vi "대한상공회의소 데이터셋 모으기(SM).vi"() -> ()   [LabVIEW 2020]
uses:
  <vilib>/DAQmx/read.llb/DAQmx Read (Analog 1D Wfm NChan NSamp).vi
  <vilib>/Analysis/baseanly.llb/Mean (DBL).vi
  <vilib>/DAQmx/create/channels.llb/DAQmx Create Channel (AI-Voltage-Basic).vi
  <vilib>/DAQmx/configure/timing.llb/DAQmx Timing (Sample Clock).vi
  <vilib>/DAQmx/miscellaneous.llb/DAQmx Fill In Error Info.vi
  <vilib>/Utility/file.llb/Write Delimited Spreadsheet (DBL).vi
  <vilib>/Analysis/NI_AALBase.lvlib
panel:
  in  "저장":bool
  out "결과":string
  out "출력 클러스터":cluster{dbl, dbl, dbl, dbl}(graph)
  in  "정지":bool
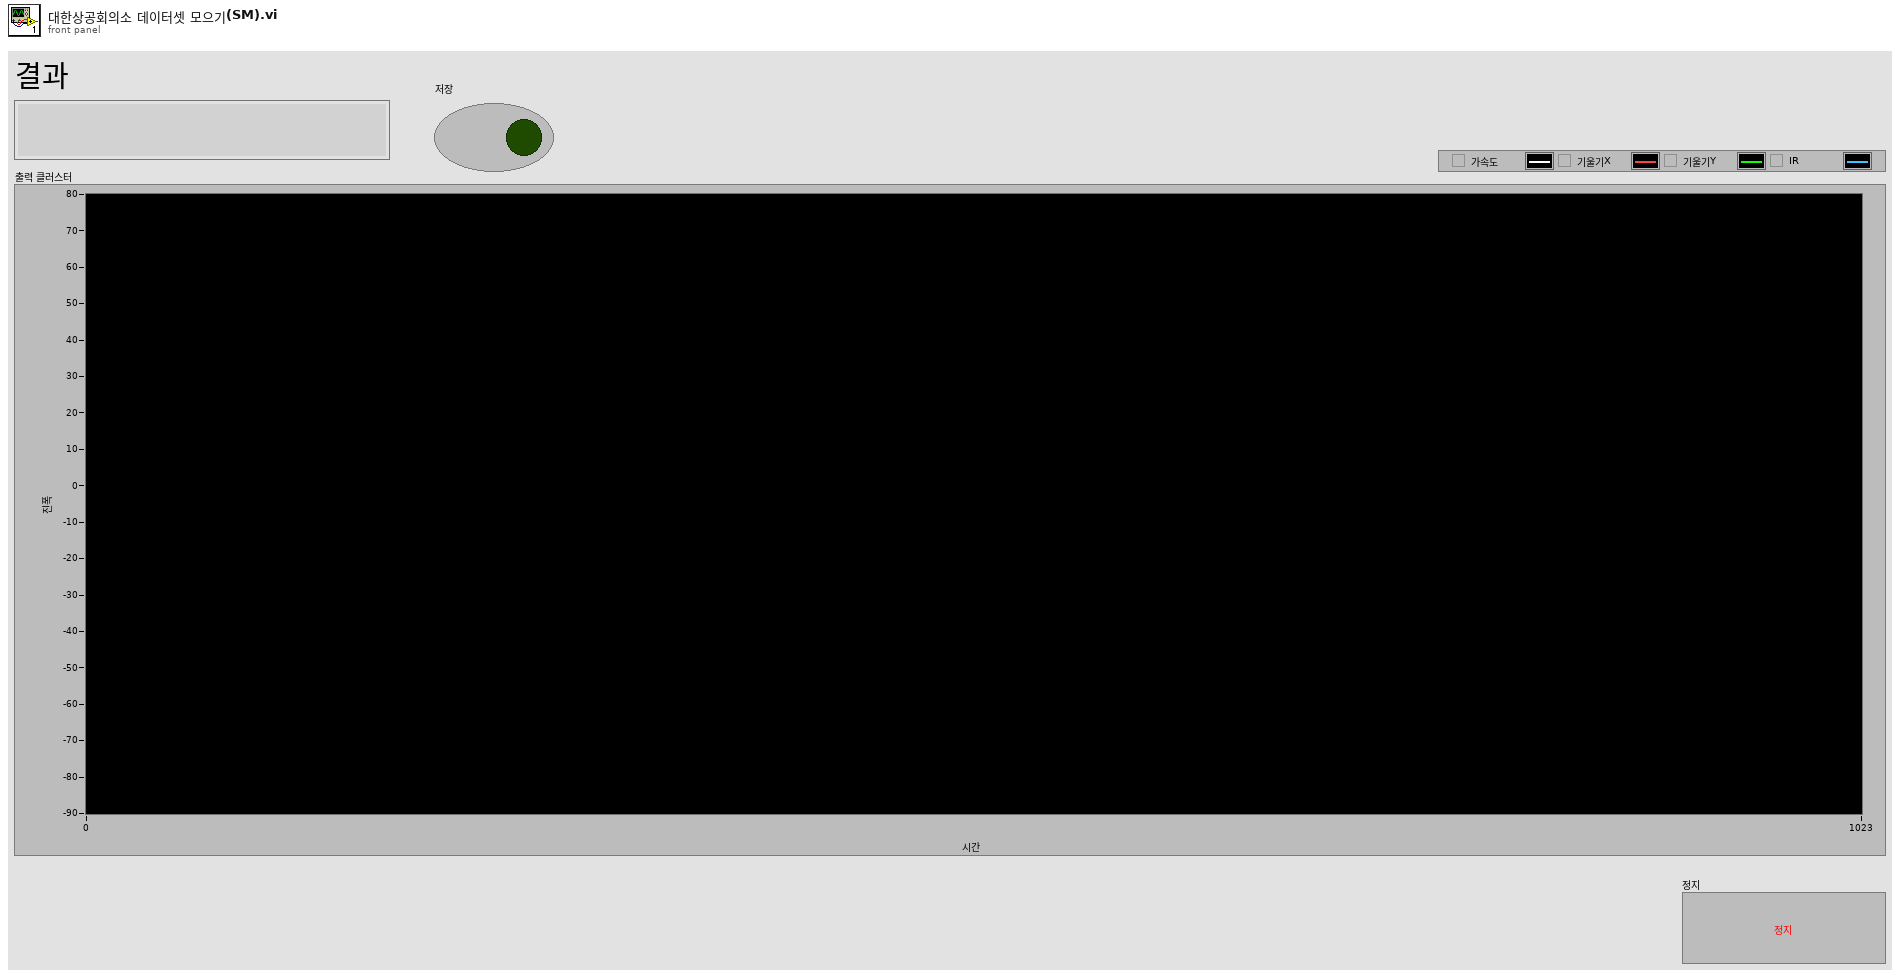
[diagram p1: front panel]
types:
  T1 = cluster{"mean":dbl, "mean":dbl, "mean":dbl, "mean":dbl}
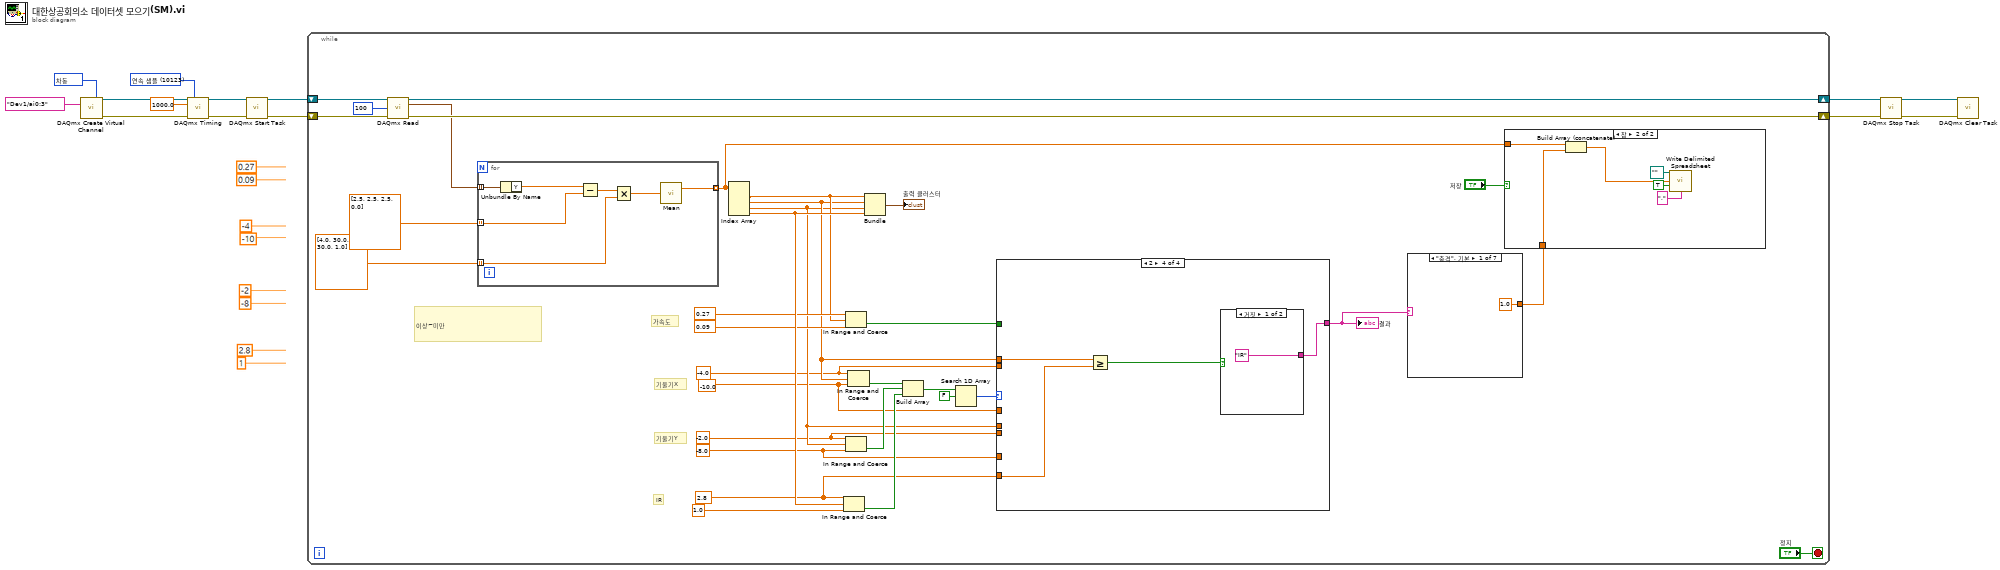
[diagram p0: block diagram]
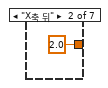
[diagram p3: hidden frame]
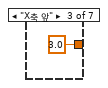
[diagram p4: hidden frame]
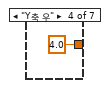
[diagram p5: hidden frame]
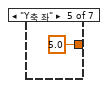
[diagram p6: hidden frame]
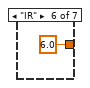
[diagram p7: hidden frame]
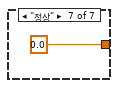
[diagram p8: hidden frame]
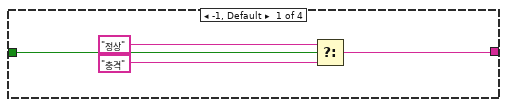
[diagram p9: hidden frame]
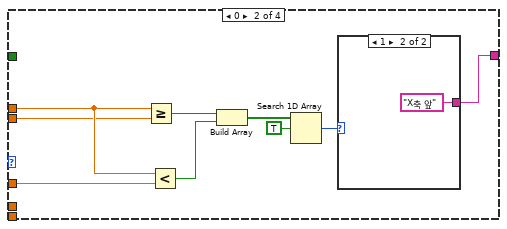
[diagram p10: hidden frame]
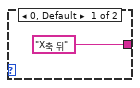
[diagram p11: hidden frame]
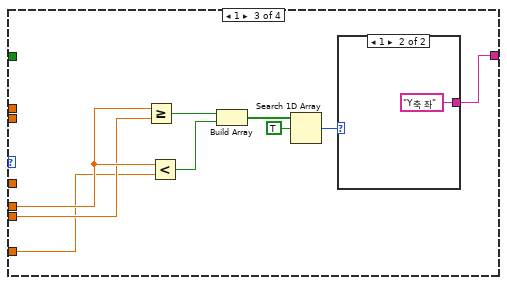
[diagram p12: hidden frame]
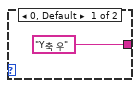
[diagram p13: hidden frame]
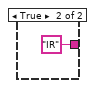
[diagram p14: hidden frame]
diagram:
  w2 = 10123 items=["유한 샘플"=10178, "연속 샘플"=10123, "하드웨어 타이밍에 의한 단일 포인트"=12522] ("sample mode")
  w3 = 10106 items=["기본"=-1, "RSE"=10083, "NRSE"=10078, "차동"=10106, "유사 차동"=12529] ("input terminal configuration")
  n1 = call-poly <vilib>:"DAQmx Create Virtual Channel.vi"("input terminal configuration"=w3, "physical channels"=tag "Dev1/ai0:3") -> ("task out"=w14:refnum<k21>, "error out"=w13:errorcluster)  [unwired: 12 in]
  n2 = call-poly <vilib>:"DAQmx Timing.vi"("task/channels in"=w14, "sample mode"=w2, "rate"=1000.0, "error in"=w13) -> ("task out"=w12:refnum<k21>, "error out"=w11:errorcluster)  [unwired: 10 in]
  n3 = call <vilib>:"DAQmx Start Task.vi"("task/channels in"=w12, "error in"=w11) -> ("task out"=w10:refnum<k21>, "error out"=w9:errorcluster)  [unwired: 12 in]
  n4 = while {
    shift-right: [w45] -> w8
    shift-left: w10 -> [w47]
    shift-right: [w44] -> w7
    shift-left: w9 -> [w46]
    stop <- "정지" stop-if-true
    w19 = 2.8 ("상위 리미트")
    w22 = -10.0 ("하위 리미트")
    w23 = -4.0 ("상위 리미트")
    w20 = -8.0 ("하위 리미트")
    w21 = -2.0 ("상위 리미트")
    # "이상~미만"
    # "IR"
    # "기울기Y"
    # "기울기X"
    # "가속도"
    n5 = call-poly <vilib>:"DAQmx Read.vi"("task/channels in"=w47, "number of samples per channel"=100, "error in"=w46) -> ("task out"=w45:refnum<k21>, "data"=w40:waveform(dbl)[], "error out"=w44:errorcluster)  [unwired: 10 in]
    n6 = for {
      tunnel: w40 -> [w99] mode=indexing
      tunnel: dbl[] [2.5, 2.5, 2.5, 0.0] -> [w97] mode=indexing
      tunnel: dbl[] [4.0, 30.0, 30.0, 1.0] -> [w96] mode=indexing
      tunnel: [w93] -> w17 mode=indexing
      n7 = Unbundle By Name(w99) -> ("Y"=w95:dbl[])
      n8 = Subtract(x=w95, y=w97) -> (x-y=w98:dbl[])
      n9 = Multiply(x=w98, y=w96) -> (x*y=w94:dbl[])
      n10 = call-poly <vilib>:"Mean.vi"("X"=w94) -> ("mean"=w93:dbl)  [unwired: 1 out]
    }
    n11 = Index Array(array=w17) -> (element #1=w29:dbl, element #2=w27:dbl, element #3=w26:dbl, element #4=w38:dbl)  [unwired: 4 in]
    n12 = In Range and Coerce(upper limit=w19, x=w38, lower limit=1.0 ("하위 리미트")) -> (In Range?=w35:bool)  [unwired: 1 out]
    n13 = In Range and Coerce(upper limit=0.27 ("상위 리미트"), x=w29, lower limit=0.09 ("하위 리미트")) -> (In Range?=w28:bool)  [unwired: 1 out]
    n14 = In Range and Coerce(upper limit=w21, x=w26, lower limit=w20) -> (In Range?=w36:bool)  [unwired: 1 out]
    n15 = In Range and Coerce(upper limit=w23, x=w27, lower limit=w22) -> (In Range?=w37:bool)  [unwired: 1 out]
    n16 = Bundle("mean"=w29, "mean"=w27, "mean"=w26, "mean"=w38) -> (→"출력 클러스터":T1)  [unwired: 1 in]
    n17 = Build Array(w37, w36, w35) -> (w34:bool[])
    n18 = Search 1D Array(1D array=w34, element=FALSE ("원소")) -> (index of element=w32:i32)  [unwired: 1 in]
    n19 = case shown="2" w32 {
      tunnel: w28 -> [w64 _ _ _]
      tunnel: [w61 w68 w79 w89] -> w18
      tunnel: w27 -> [_ w67 _ w90]
      tunnel: w26 -> [_ _ w78 _]
      tunnel: w23 -> [_ w66 _ _]
      tunnel: w22 -> [_ w65 _ _]
      tunnel: w21 -> [_ _ w77 _]
      tunnel: w20 -> [_ _ w76 _]
      tunnel: w19 -> [_ _ _ w87]
      frame -1, Default {
        n20 = Select(t="정상", s=w64, f="충격") -> (s? t:f=w61:string)
      }
      frame 0 {
        n21 = Greater Or Equal?(x=w67, y=w66) -> (x >= y?=w73:bool)
        n22 = Less?(x=w67, y=w65) -> (x < y?=w72:bool)
        n23 = Build Array(w73, w72) -> (w71:bool[])
        n24 = Search 1D Array(1D array=w71, element=TRUE ("원소")) -> (index of element=w69:i32)  [unwired: 1 in]
        n25 = case shown="1" w69 {
          tunnel: ["X축 뒤" "X축 앞"] -> w68
          frame 0, Default {
          }
          frame 1 {
          }
        }
      }
      frame 1 {
        n26 = Greater Or Equal?(x=w78, y=w77) -> (x >= y?=w84:bool)
        n27 = Less?(x=w78, y=w76) -> (x < y?=w83:bool)
        n28 = Build Array(w84, w83) -> (w82:bool[])
        n29 = Search 1D Array(1D array=w82, element=TRUE ("원소")) -> (index of element=w80:i32)  [unwired: 1 in]
        n30 = case shown="1" w80 {
          tunnel: ["Y축 우" "Y축 좌"] -> w79
          frame 0, Default {
          }
          frame 1 {
          }
        }
      }
      frame 2 {
        n31 = Greater Or Equal?(x=w90, y=w87) -> (x >= y?=w88:bool)
        n32 = case shown="거짓" w88 {
          tunnel: ["IR" "IR"] -> w89
          frame False {
          }
          frame True {
          }
        }
      }
    }
    "결과" <- w18
    n33 = case shown="\"충격\", 기본" w18 {
      tunnel: [1.0 2.0 3.0 4.0 5.0 6.0 0.0] -> w16
      frame "충격", Default {
      }
      frame "X축 뒤" {
      }
      frame "X축 앞" {
      }
      frame "Y축 우" {
      }
      frame "Y축 좌" {
      }
      frame "IR" {
      }
      frame "정상" {
      }
    }
    n34 = case shown="참" "저장" {
      tunnel: w17 -> [_ w53]
      tunnel: w16 -> [_ w52]
      frame False {
      }
      frame True {
        n35 = Build Array (concatenate)(w53, w52) -> (w51:dbl[])
        n36 = call-poly <vilib>:"Write Delimited Spreadsheet.vi"("file path (dialog if empty)"=path "", "1D data"=w51, "append to file? (new file:F)"=TRUE, "delimiter (\\t)"="," ("delimiter (\\t)")) -> ()  [unwired: 10 in, 2 out]
      }
    }
  }
  n37 = call <vilib>:"DAQmx Stop Task.vi"("task/channels in"=w8, "error in"=w7) -> ("task out"=w6:refnum<k21>, "error out"=w5:errorcluster)  [unwired: 12 in]
  n38 = call <vilib>:"DAQmx Clear Task.vi"("task in"=w6, "error in"=w5) -> ()  [unwired: 13 in, 1 out]
